vi "Map Control Message.vi"(11 "Pump Controls":T1) -> (1 "Control Message":dbl[](array[numeric]))   [LabVIEW 2025, in "phlair-busch-can-bus.lvlib"]
uses:
  phlair-busch-can-bus.lvlib
  PumpControls.ctl
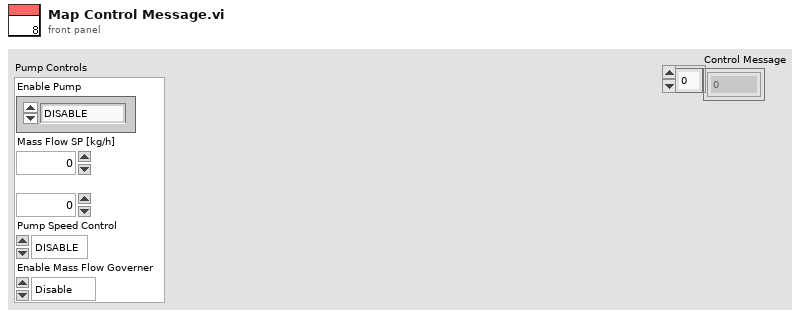
[diagram p1: front panel]
types:
  T1 = typedef "phlair-busch-can-bus.lvlib/PumpControls.ctl" = cluster{"Enable Pump":enum16{"DISABLE", "ENABLE"}, "Mass Flow SP [kg/h]":dbl, "Speed SP [U/ min]":u16, "Pump Speed Control":enum16{"DISABLE", "ENABLE"}, "Enable Mass Flow Governer":enum8{"Disable", "Enable", "", "NA"}}
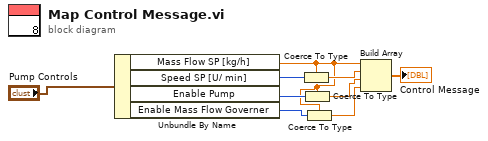
[diagram p0: block diagram]
diagram:
  n1 = Unbundle By Name("Pump Controls") -> ("Mass Flow SP [kg/h]"=w3:dbl, "Speed SP [U/ min]"=w8:u16, "Enable Pump"=w7:enum16{"DISABLE", "ENABLE"}, "Enable Mass Flow Governer"=w4:enum8{"Disable", "Enable", "", "NA"})
  n2 = Coerce To Type(0:w8, 1:w3) -> (2:w6:dbl)
  n3 = Coerce To Type(0:w7, 1:w3) -> (2:w5:dbl)
  n4 = Coerce To Type(0:w4, 1:w3) -> (2:w2:dbl)
  n5 = Build Array(w3, w6, w5, w2) -> (→"Control Message":dbl[])
